vi "New ApplicationEventHandler.vi"(6 "EventFilter Reference":T1, 7 "Timeout Message Priority (Normal)":T2=enum."Normal", 8 "Timeout [ms]":i32=-1, 9 "Timeout Message":refnum<class "RoundTripMessage.lvclass">, 10 "Registrations":T3[](array[typedef])) -> (0 "error out":errorcluster, 3 "ApplicationEventHandler":refnum<class "ApplicationEventHandler.lvclass">)   [LabVIEW 2020, in "ActorEvents.lvlib" / "ApplicationEventHandler.lvclass"]
uses:
  ApplicationEventHandler.lvclass
  ApplicationEventHandler.lvclass/ApplicationEventHandler.ctl
  IEventHandler/IEventHandler.lvclass
  C:/Git/mva-viewable/Source/ActorEvents/IEventHandler/IEventHandler.lvclass
  C:/Program Files (x86)/National Instruments/LabVIEW 2020/vi.lib/ActorFramework/Actor/Actor.lvclass
  C:/Git/mva-viewable/Source/ActorEvents/EventHandler/ApplicationEventHandler/ApplicationEventHandler.lvclass
  composed-af-messages/Source/RoundTripMessage/RoundTripMessage.lvclass
  C:/Program Files (x86)/National Instruments/LabVIEW 2020/vi.lib/ActorFramework/Message/Message.lvclass
  C:/Git/mva-viewable/modules/composed-af-messages/Source/RoundTripMessage/RoundTripMessage.lvclass
  <vilib>/event_ctls.llb/lveventtype.ctl
  <vilib>/ActorFramework/Message Enqueuer/Message Priority.ctl
  <vilib>/ActorFramework/Message Enqueuer/Message Enqueuer.lvclass
  IEventFilter/IEventFilter.lvclass
  IEventFilter/EventFilter Reference.ctl
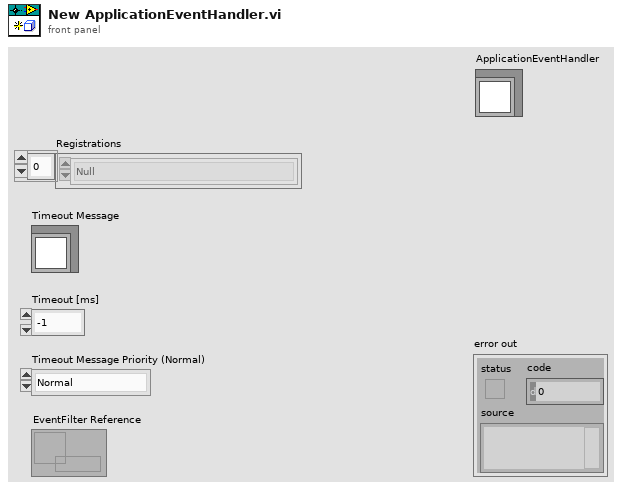
[diagram p1: front panel]
types:
  T1 = typedef "ActorEvents.lvlib/IEventFilter.lvclass/EventFilter Reference.ctl" = refnum<data-value>
  T2 = typedef "Actor Framework.lvlib/Message Enqueuer.lvclass/Message Priority.ctl" = enum16{"Low", "Normal", "High"}
  T3 = typedef "lveventtype.ctl" = enum32{"Null", "Timeout", "Annotation Menu Selection", "Annotation Menu Selection?", "App Instance Close", "App Instance Close?", "Autoscale Range Change", "Bookmark Info Change", "Cell Edit", "Cell Edit?", "Cursor Grab", "Cursor Grab?", "Cursor Menu Selection", "Cursor Menu Selection?", "Cursor Move", "Cursor Release", "Data Change", "Direction Change", "Display State Change", "Drag Ended", "Drag Enter", "Drag Leave", "Drag Over", "Drag Source Update", "Drag Starting", "Drag Starting?", "Drop", "Exec State Change", "Key Down", "Key Down?", "Key Repeat", "Key Repeat?", "Key Up", "Listbox Double Click", "Menu Activation?", "Menu Selection (App)", "Menu Selection? (App)", "Menu Selection (User)", "Mouse Down", "Mouse Down?", "Mouse Enter", "Mouse Leave", "Mouse Move", "Mouse Up", "Mouse Wheel", "NI Security User Change (App)", "Pane Size", "Panel Close", "Panel Close?", "Panel Resize", "Plot Attribute Change", "Scale Range Change", "Shortcut Menu Activation?", "Shortcut Menu Selection (App)", "Shortcut Menu Selection? (App)", "Shortcut Menu Selection (User)", "Tree Double Click", "Tree Drag", "Tree Drag?", "Tree Drop", "Tree Drop?", "Tree Item Close", "Tree Item Close?", "Tree Item Open", "Tree Item Open?", "User Event", "Value Change"}
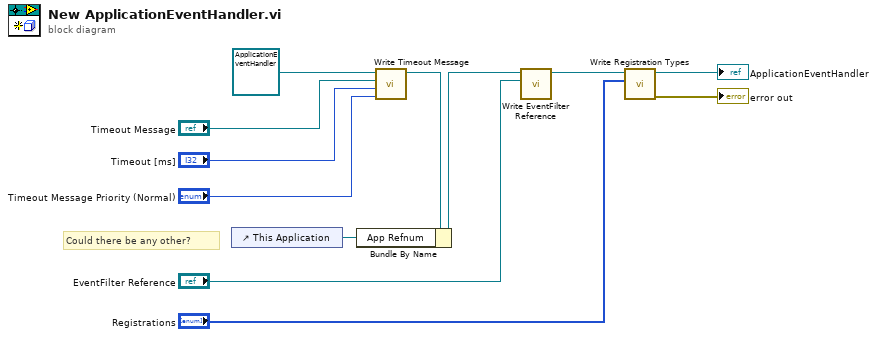
[diagram p0: block diagram]
diagram:
  # "Could there be any other?"
  n1 = control-ref of="This Application"() -> (w7:refnum<vi>)
  n2 = call "Write Timeout Message.vi"("Timeout Message Priority (Normal)"="Timeout Message Priority (Normal)", "Timeout [ms]"="Timeout [ms]", "Timeout Message"="Timeout Message", "IEventHandler in"=refnum<class "ApplicationEventHandler.lvclass"> refnum ("ApplicationEventHandler In")) -> ("IEventHandler out"=w11:refnum<class "ApplicationEventHandler.lvclass">)  [unwired: 7 in]
  n3 = Bundle By Name(cluster=w11, "App Refnum"=w7) -> (w12:refnum<class "ApplicationEventHandler.lvclass">)
  n4 = call "Write EventFilter Reference.vi"("EventFilter Reference"="EventFilter Reference", "IEventHandler in"=w12) -> ("IEventHandler out"=w2:refnum<class "ApplicationEventHandler.lvclass">)  [unwired: 9 in]
  n5 = call "Write Registration Types.vi"("Requested Registration Types"="Registrations", "IEventHandler In"=w2) -> ("error out"=→"error out":errorcluster, "IEventHandler Out"=→"ApplicationEventHandler":refnum<class "ApplicationEventHandler.lvclass">)  [unwired: 8 in]
